vi "Write-Completo.vi"(5 "Low Byte":string, 6 "Dato 8 bits":string, 7 "Hi Byte":string, 8 "error in (no error)":errorcluster, 11 "VISA resource name":refnum<visa-resource-name>) -> (0 "error out":errorcluster, 3 "VISA resource name out":refnum<visa-resource-name>)   [LabVIEW 2014, in "CAP-USB.lvlib"]
doc: "Ennvia el comando de escritura al CAP-USB, \nHi Byte, Low Byte, determinan la direccion en la que se \nva a escribir"
uses:
  CAP-USB.lvlib
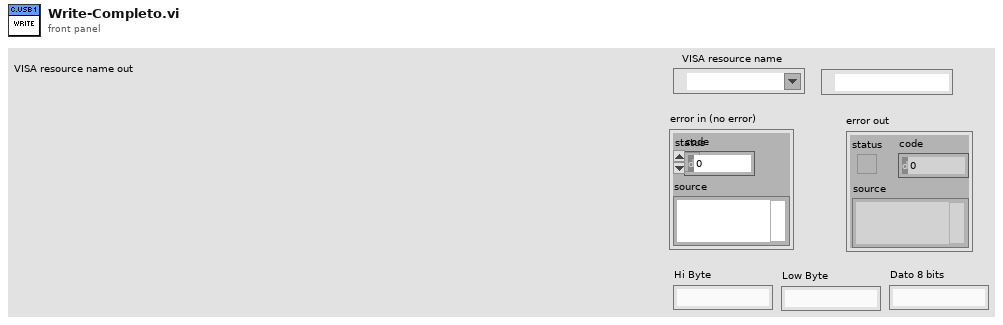
[diagram p1: front panel]
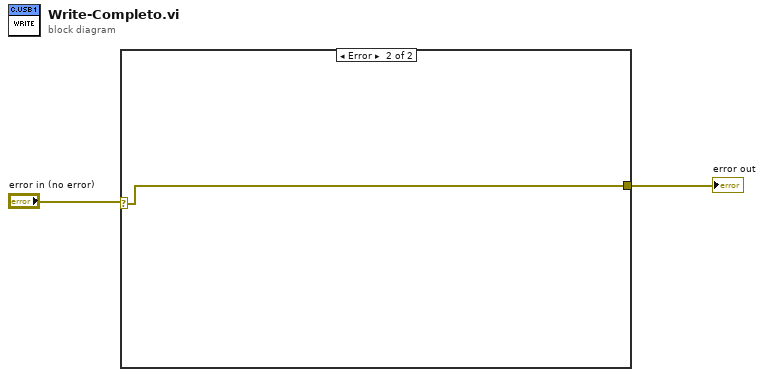
[diagram p0: block diagram]
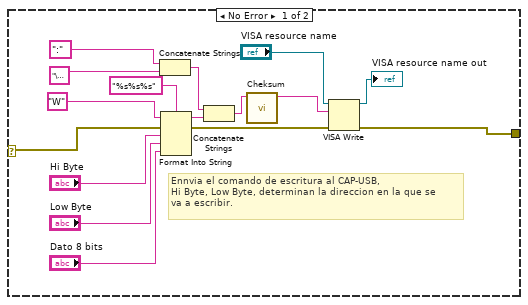
[diagram p2: hidden frame]
diagram:
  n1 = case shown="Error" "error in (no error)" {
    selector: "error in (no error)" -> [w3 w19]
    tunnel: [w14 w19] -> w2
    frame No Error {
      # "Ennvia el comando de escritura al CAP-USB, \nHi Byte, Low Byte, determinan la direccion en la que se \nva a escribir."
      n2 = Concatenate Strings(":" ("COMANDO (e)"), "\u0004" ("COMANDO (e)")) -> (w7:string)
      n3 = Format Into String(format string="%s%s%s", initial string="W" ("WRITE(W)"), error in=w3, "Hi Byte", "Low Byte", "Dato 8 bits") -> (resulting string=w6:string, error out=w18:errorcluster)
      n4 = Concatenate Strings(w7, w6) -> (w5:string)
      n5 = call "Cheksum.vi"("Trama IN"=w5) -> ("Trama RTS"=w4:string)  [unwired: 9 in, 1 out]
      n6 = VISA Write(VISA resource name="VISA resource name", write buffer=w4, error in (no error)=w18) -> (VISA resource name out=→"VISA resource name out":refnum<visa-resource-name>, error out=w14:errorcluster)  [unwired: 1 out]
    }
    frame Error {
    }
  }
  "error out" <- w2
